vi "DS345_BurstMode.get gate.vi"(0 "i ref in":refnum<vi>, 5 "error in (no error)":errorcluster) -> (14 "i ref out":refnum<vi>, 16 "gate [us]":dbl format="%.2f", 19 "error out":errorcluster)   [LabVIEW 2014, in "DS345_BurstMode.lvlib"]
doc: "gets the value for the gate (pulse width) that is to be used when calling the \"set delay\" method."
uses:
  DS345_BurstMode.lvlib
  CSCore/BaseProcess/BaseProcess.lvlib
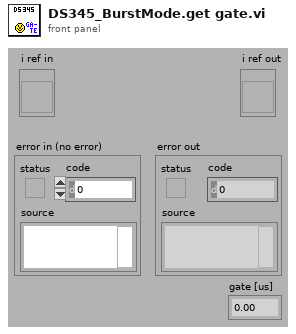
[diagram p1: front panel]
types:
  T1 = typedef "BaseProcess.lvlib/BaseProcess.i attribute.ctl" = cluster{"EventStatus":string, "EventError":i32, "PresetEvtWatchD":i32, "PresetPdcWatchD":i32, "EventTimeout":i32, "PeriodicInterval":i32, "Interface":string[], "Address":string[], "Special":string[], "PeriodicError":i32, "PeriodicStatus":string, "SuperProc":string, "Descriptors":T2[], "CaseRef":refnum<vi>, "PdcRef":refnum<vi>, "Thread Ref":refnum<vi>, "eventErrorID":i32, "eventStatusID":i32, "periodicErrorID":i32, "periodicStatusID":i32, "pdcCtrID":i32}
  T2 = typedef "BaseProcess.lvlib/BaseProcess.descriptor definition.ctl" = cluster{"selector":string, "descriptor":T3}
  T3 = typedef "BaseProcess.lvlib/BaseProcess.descriptor string definition.ctl" = string
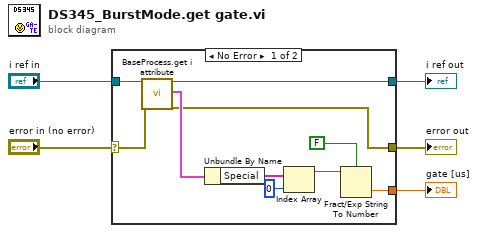
[diagram p0: block diagram]
diagram:
  n1 = case shown="No Error" "error in (no error)" {
    selector: "error in (no error)" -> [w7 w16]
    tunnel: "i ref in" -> [w15 w17]
    tunnel: [w10 _] -> w4
    tunnel: [w9 w17] -> w3
    tunnel: [w8 w16] -> w2
    frame No Error {
      n2 = call "BaseProcess.get i attribute.vi"("i ref in"=w15, "error in (no error)"=w7) -> ("i ref out"=w9:refnum<vi>, "i attribute"=w14:T1, "error out"=w8:errorcluster)  [unwired: 15 in]
      n3 = Unbundle By Name(w14) -> ("Special"=w13:string[])
      n4 = Index Array(array=w13, index=0 ("Index")) -> (element=w11:string)
      n5 = Fract/Exp String To Number(use system decimal point (T)=FALSE, string=w11) -> (number=w10:dbl)  [unwired: 2 in, 1 out]
    }
    frame Error {
    }
  }
  "error out" <- w2
  "i ref out" <- w3
  "gate [us]" <- w4
